vi "Tx_Rx_Log.vi"(0 "VISA in":refnum<visa-resource-name>, 1 "Timeout (3000)":i32=3000, 2 "Log?":bool, 5 "Fbk? (T)":bool=TRUE, 9 "Write":string, 11 "error in":errorcluster, 12 "TermChar (\\n)":string="\n", 13 "Wait for? (\\n)":string="\n") -> (3 "ExecTime(ms)":i32, 4 "VISA out":refnum<visa-resource-name>, 6 "Timeout?":bool, 10 "Read":string, 15 "error out":errorcluster)   [LabVIEW 2016, in "Serial_G.lvlib"]
doc: "Sends, reads and logs VISA command"
uses:
  Serial_G.lvlib
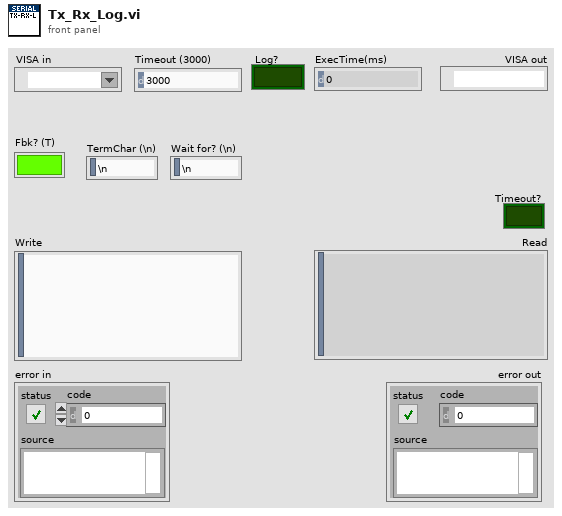
[diagram p1: front panel]
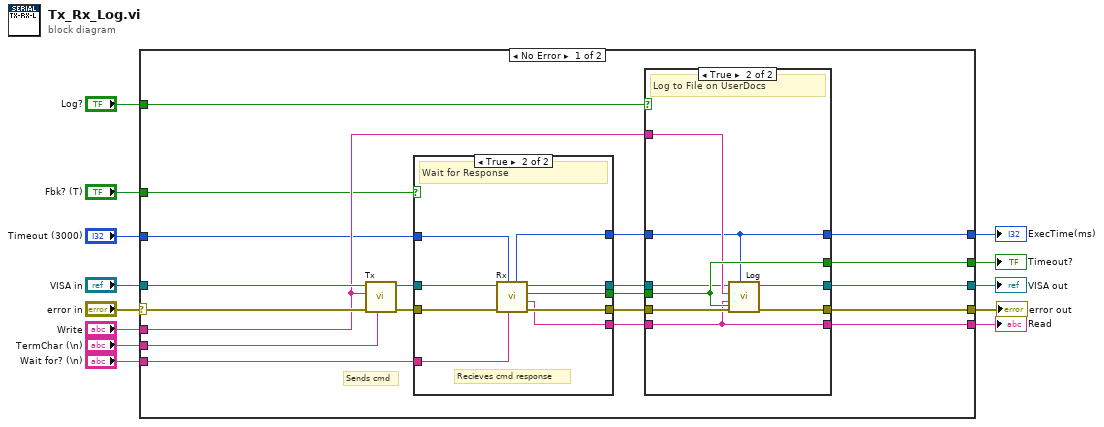
[diagram p0: block diagram]
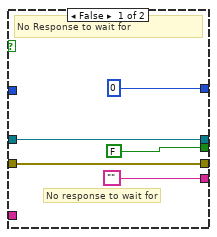
[diagram p3: hidden frame]
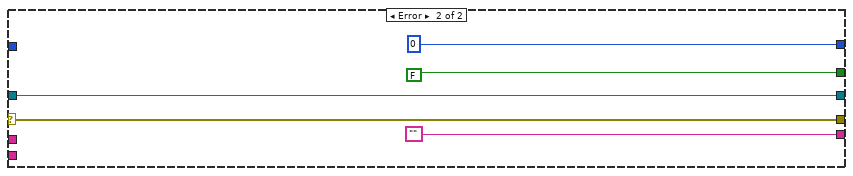
[diagram p4: hidden frame]
diagram:
  n1 = case shown="No Error" "error in" {
    selector: "error in" -> [w31 w65]
    tunnel: [w29 w65] -> w12
    tunnel: "Wait for? (\\n)" -> [w24 _]
    tunnel: "VISA in" -> [w23 w64]
    tunnel: "Write" -> [w22 _]
    tunnel: "Timeout (3000)" -> [w21 _]
    tunnel: "Fbk? (T)" -> [w20 _]
    tunnel: "Log?" -> [w19 _]
    tunnel: "TermChar (\\n)" -> [w18 _]
    tunnel: [w17 0] -> w4
    tunnel: [w16 FALSE] -> w3
    tunnel: [w15 w64] -> w2
    tunnel: [w14 ""] -> w1
    frame No Error {
      # "Sends cmd"
      n2 = call "Tx.vi"("TermChar (\\r\\n)"=w18, "error in"=w31, "Command"=w22, "VISA in"=w23) -> ("error out"=w32:errorcluster, "VISA out"=w33:refnum<visa-resource-name>)  [unwired: 6 in]
      n3 = case shown="True" w20 {
        tunnel: w33 -> [w51 w60]
        tunnel: w32 -> [w49 w59]
        tunnel: w21 -> [_ w56]
        tunnel: [w49 w58] -> w30
        tunnel: [0 ("Time (ms)") w55] -> w27
        tunnel: w24 -> [_ w52]
        tunnel: [w51 w57] -> w25
        tunnel: [FALSE ("Timeout?") w54] -> w26
        tunnel: ["" w53] -> w28
        frame False {
          # "No response to wait for"
          # "No Response to wait for"
        }
        frame True {
          # "Recieves cmd response"
          # "Wait for Response"
          n4 = call "Rx.vi"("Wait for? (\\r\\n)"=w52, "Timeout_ms (3000)"=w56, "error in"=w59, "VISA in"=w60) -> ("error out"=w58:errorcluster, "Response"=w53:string, "Timeout?"=w54:bool, "VISA out"=w57:refnum<visa-resource-name>, "ExecTime(ms)"=w55:i32)  [unwired: 3 in]
        }
      }
      n5 = case shown="True" w19 {
        tunnel: w30 -> [w34 w46]
        tunnel: [w34 w45] -> w29
        tunnel: w22 -> [_ w42]
        tunnel: w28 -> [w37 w43]
        tunnel: w27 -> [w36 w39]
        tunnel: w26 -> [w35 w44]
        tunnel: [w38 w40] -> w15
        tunnel: w25 -> [w38 w41]
        tunnel: [w37 w43] -> w14
        tunnel: [w36 w39] -> w17
        tunnel: [w35 w44] -> w16
        frame False {
          # "No Log"
        }
        frame True {
          # "Log to File on UserDocs"
          n6 = call "Log.vi"("Timeout"=w44, "ExecTime (ms)"=w39, "error in"=w46, "Response"=w43, "Command"=w42, "VISA in"=w41) -> ("error out"=w45:errorcluster, "VISA out"=w40:refnum<visa-resource-name>)  [unwired: 3 in, 1 out]
        }
      }
    }
    frame Error {
    }
  }
  "error out" <- w12
  "Read" <- w1
  "VISA out" <- w2
  "Timeout?" <- w3
  "ExecTime(ms)" <- w4
